vi "Update Data.vi"(8 "error in (no error)":errorcluster, 10 "Data Point":dbl, 11 "Report in":refnum<class "Wind TXT Report.lvclass">) -> (0 "error out":errorcluster, 3 "Report out":refnum<class "Wind TXT Report.lvclass">)   [LabVIEW 2009, in "Wind TXT Report.lvclass"]
doc: "This VI is a dynamic dispatch that overrides the parent method.\n\nAAL 9/09"
uses:
  Wind TXT Report.lvclass
  Wind Report/Wind Report.lvclass
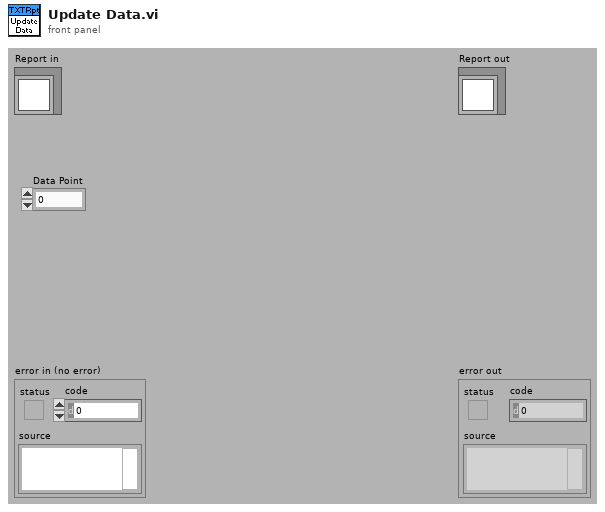
[diagram p1: front panel]
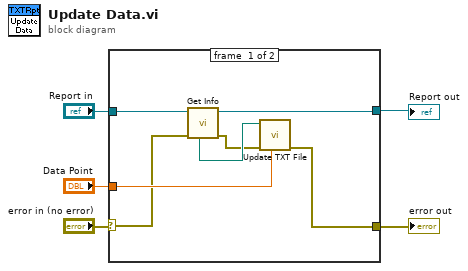
[diagram p0: block diagram]
diagram:
  n1 = case shown="No Error" "error in (no error)" {
    selector: "error in (no error)" -> [w8 w13]
    tunnel: "Report in" -> [w7 w14]
    tunnel: "Data Point" -> [w11 _]
    tunnel: [w9 w13] -> w3
    tunnel: [w6 w14] -> w1
    frame #0 {
      n2 = call "Get Info.vi"("error in (no error)"=w8, "Report.lvclass in"=w7) -> ("error out"=w10:errorcluster, "Report.lvclass out"=w6:refnum<class "Wind TXT Report.lvclass">, "Path"=w12:path)  [unwired: 3 in, 4 out]
      n3 = call "Update TXT File.vi"("Data Point"=w11, "error in"=w10, "Path"=w12) -> ("error out"=w9:errorcluster)  [unwired: 8 in]
    }
    frame #1 {
    }
  }
  "error out" <- w3
  "Report out" <- w1
